vi "ramping.vi"(10 "Speed":dbl, 11 "Max Change":dbl) -> (3 "New Speed":dbl)   [LabVIEW 2014]
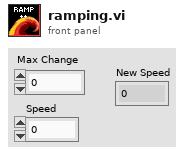
[diagram p1: front panel]
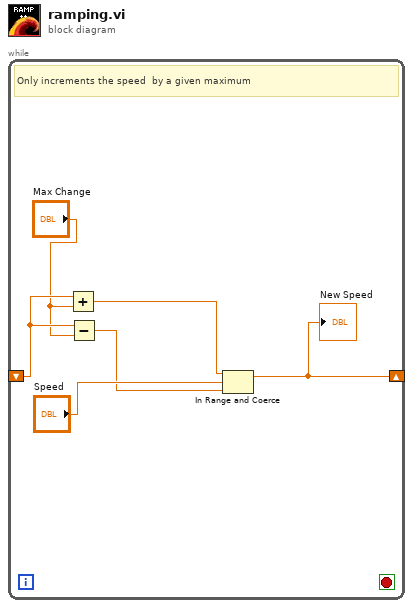
[diagram p0: block diagram]
diagram:
  n1 = while {
    shift-right: [w5] -> _
    shift-left: _ -> [w2]
    stop <- _ stop-if-true
    # "Only increments the speed  by a given maximum"
    n2 = Add(x=w2, y="Max Change") -> (x+y=w4:dbl)
    n3 = Subtract(x=w2, y="Max Change") -> (x-y=w3:dbl)
    n4 = In Range and Coerce(upper limit=w4, x="Speed", lower limit=w3) -> (coerced(x)=w5:dbl)  [unwired: 1 out]
    "New Speed" <- w5
  }
